vi "Practica_11_Amplitud_Modulada_Save_TXT.vi"() -> ()   [LabVIEW 2016]
panel:
  in  "Save Data?":bool
  in  "Muestras":i32(slide) scale=0.0..1000.0
  in  "Amplitud Info":dbl(knob) scale=0.0..10.0
  in  "Frecuencia Info":dbl(knob) scale=0.0..10.0
  in  "Amplitud Carrier":dbl(knob) scale=0.0..100.0
  in  "Frecuencia Carrier":dbl(knob) scale=0.0..100.0
  out "Waveform Graph":dbl[](graph)
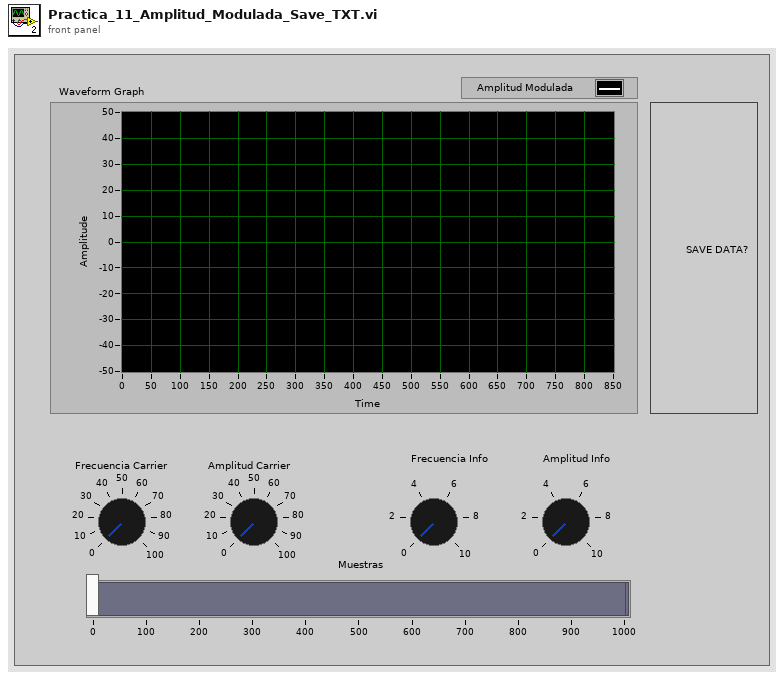
[diagram p1: front panel]
types:
  T1 = enum16{"open", "replace", "create", "open or create", "replace or create", "replace or create with confirmation"}
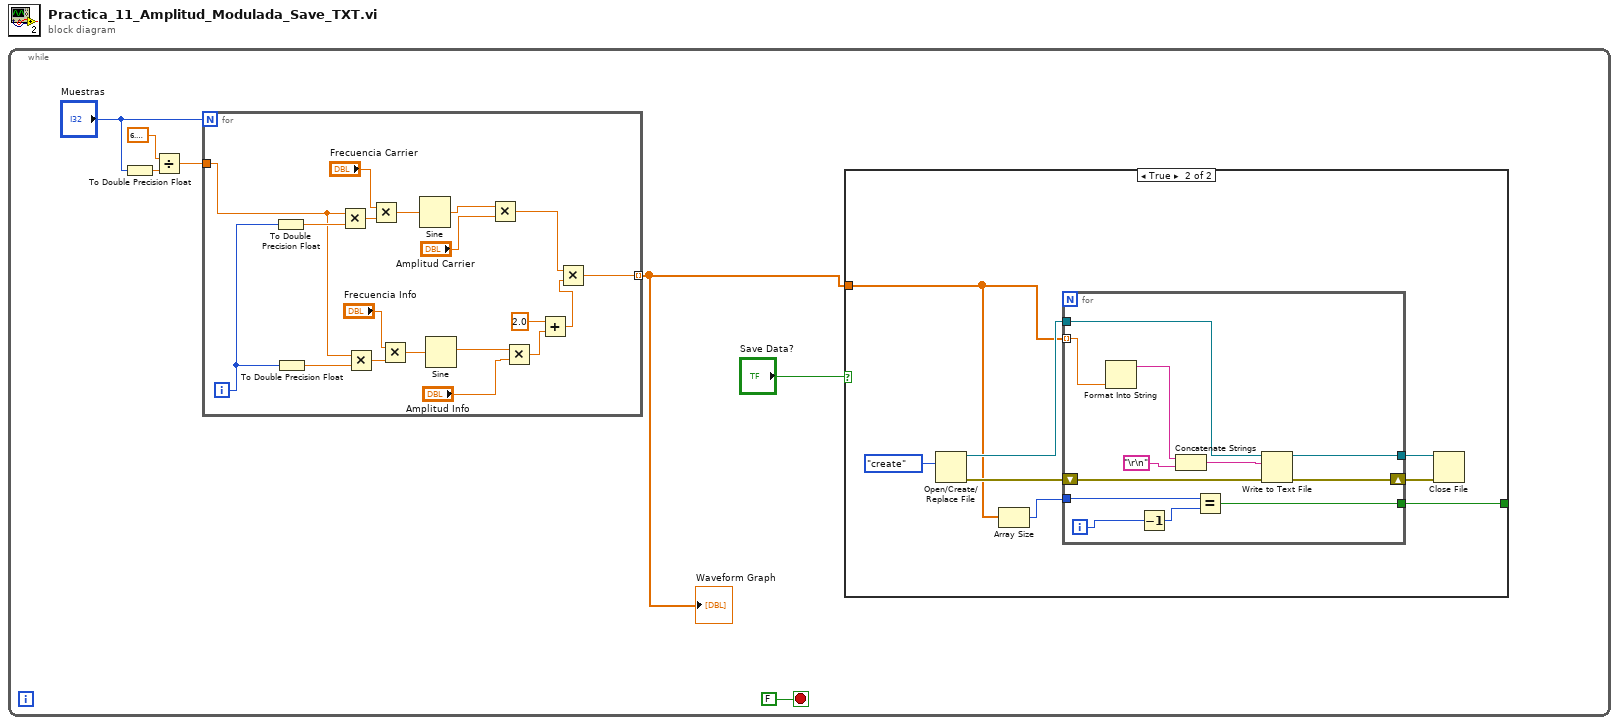
[diagram p0: block diagram]
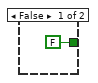
[diagram p2: hidden frame]
diagram:
  n1 = while {
    stop <- FALSE stop-if-true
    n2 = To Double Precision Float(number="Muestras") -> (double precision float=w6:dbl)
    n3 = Divide(x=6.283185307179586, y=w6) -> (x/y=w4:dbl)
    n4 = for {
      N: "Muestras" -> [_]
      tunnel: w4 -> [w44]
      tunnel: [w33] -> w2 mode=indexing
      i -> [w45]
      n5 = To Double Precision Float(number=w45) -> (double precision float=w47:dbl)
      n6 = To Double Precision Float(number=w45) -> (double precision float=w46:dbl)
      n7 = Multiply(x=w44, y=w47) -> (x*y=w43:dbl)
      n8 = Multiply(x=w44, y=w46) -> (x*y=w40:dbl)
      n9 = Multiply(x="Frecuencia Carrier", y=w43) -> (x*y=w41:dbl)
      n10 = Multiply(x="Frecuencia Info", y=w40) -> (x*y=w38:dbl)
      n11 = Sine(x=w41) -> (sin(x)=w36:dbl)
      n12 = Sine(x=w38) -> (sin(x)=w35:dbl)
      n13 = Multiply(x=w36, y="Amplitud Carrier") -> (x*y=w34:dbl)
      n14 = Multiply(x=w35, y="Amplitud Info") -> (x*y=w32:dbl)
      n15 = Add(x=2.0, y=w32) -> (x+y=w31:dbl)
      n16 = Multiply(x=w34, y=w31) -> (x*y=w33:dbl)
    }
    "Waveform Graph" <- w2
    n17 = case shown="True" "Save Data?" {
      tunnel: w2 -> [_ w11]
      tunnel: [FALSE w9] -> _
      frame False {
      }
      frame True {
        n18 = Open/Create/Replace File(operation (0:open)=T1."create") -> (refnum out=w13:refnum<file>, error out=w16:errorcluster)  [unwired: 5 in, 1 out]
        n19 = Array Size(array=w11) -> (size(s)=w10:i32)
        n20 = for {
          tunnel: w11 -> [w26] mode=indexing
          tunnel: w13 -> [w22]
          tunnel: [w21] -> w12
          tunnel: w10 -> [w18]
          tunnel: [w17] -> w9
          shift-right: [w27] -> w15
          shift-left: w16 -> [w28]
          i -> [w20]
          n21 = Format Into String(w26) -> (resulting string=w24:string)  [unwired: 3 in, 1 out]
          n22 = Decrement(x=w20) -> (x-1=w19:i32)
          n23 = Concatenate Strings(w24, "\r\n") -> (w23:string)
          n24 = Equal?(x=w18, y=w19) -> (x = y?=w17:bool)
          n25 = Write to Text File(file (use dialog)=w22, text=w23, error in=w28) -> (refnum out=w21:refnum<file>, error out=w27:errorcluster)  [unwired: 1 in, 1 out]
        }
        n26 = Close File(refnum=w12, error in=w15) -> ()  [unwired: 2 out]
      }
    }
  }
